vi "Get X and Y (single).vi"(8 "error in (no error)":errorcluster, 11 "XY-data":cluster{"X-array":dbl[], "Y-array":dbl[]} {"Y-array" format="%.2p"; "X-array" format="%.2p"}) -> (0 "error out":errorcluster, 1 "Y-array":dbl[](array[numeric]), 2 "X-array":dbl[](array[numeric]), 3 "XY-data out":cluster{"X-array":dbl[], "Y-array":dbl[]} {"Y-array" format="%.2p"; "X-array" format="%.2p"})   [LabVIEW 2016, in "xy_utilities.lvlib"]
doc: "Returns the X and Y arrays contained in <b>XY-data</b>.\n\nWire data to the data input to determine the polymorphic instance to use or manually select the instance."
uses:
  xy_utilities.lvlib
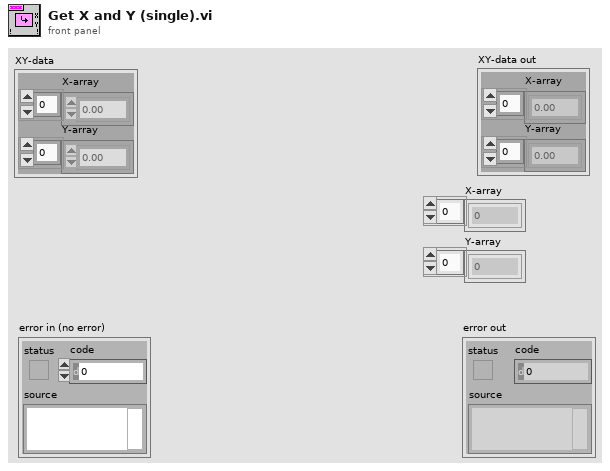
[diagram p1: front panel]
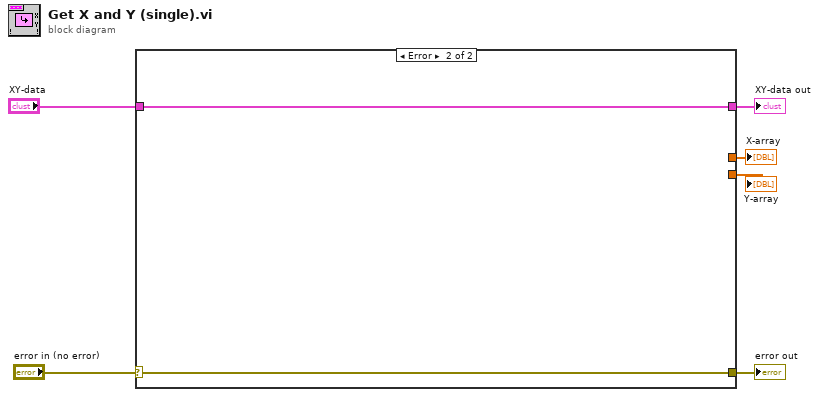
[diagram p0: block diagram]
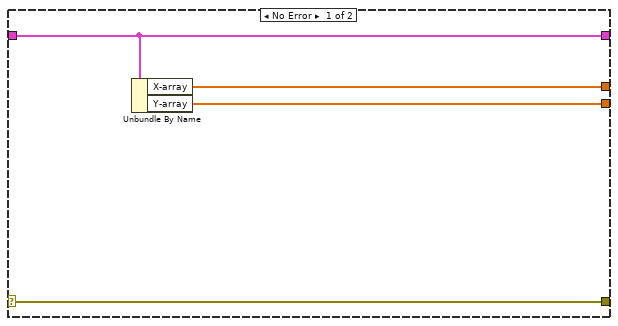
[diagram p2: hidden frame]
diagram:
  n1 = case shown="Error" "error in (no error)" {
    selector: "error in (no error)" -> [w10 w12]
    tunnel: [w10 w12] -> w5
    tunnel: "XY-data" -> [w9 w11]
    tunnel: [w9 w11] -> w3
    tunnel: [w8 _] -> w2
    tunnel: [w7 _] -> w1
    frame No Error {
      n2 = Unbundle By Name(w9) -> ("X-array"=w8:dbl[], "Y-array"=w7:dbl[])
    }
    frame Error {
    }
  }
  "error out" <- w5
  "XY-data out" <- w3
  "X-array" <- w2
  "Y-array" <- w1
